vi "SPIEngineSOM.vi"(7 "NumNodes":u8=1) -> ()   [LabVIEW 2014, in "IO Node Logic Template_SPIBus0.lvlib"]
uses:
  IO Node Logic Template_SPIBus0.lvlib
  <vilib>/SPIAPI/DIO/SPI Digital IO Lines.ctl
  <vilib>/SPIAPI/DIO/SPI DIO Enable Lines.ctl
  Node/Controls/NodeResources FIFOs.ctl
  Controls/All Nodes Resources.ctl
  <vilib>/Platform/TimedLoop/XDataNode/XDataNode.xnode
  <vilib>/Platform/TimedLoop/XDataNode/nitl_modes.ctl
  <vilib>/Platform/TimedLoop/XDataNode/XDNodeRunTimeDep.lvlib
  <vilib>/Platform/TimedLoop/XDataNode/wakeup.ctl
  <vilib>/Platform/TimedLoop/XDataNode/timing_clust.ctl
  <userlib>/_NI SPI IP/FPGA/Controllers/Public/Spi Master Outputs.ctl
  <userlib>/_NI SPI IP/FPGA/Controllers/NI SPI IP FPGA.lvlib
panel:
  out "spi output":T1
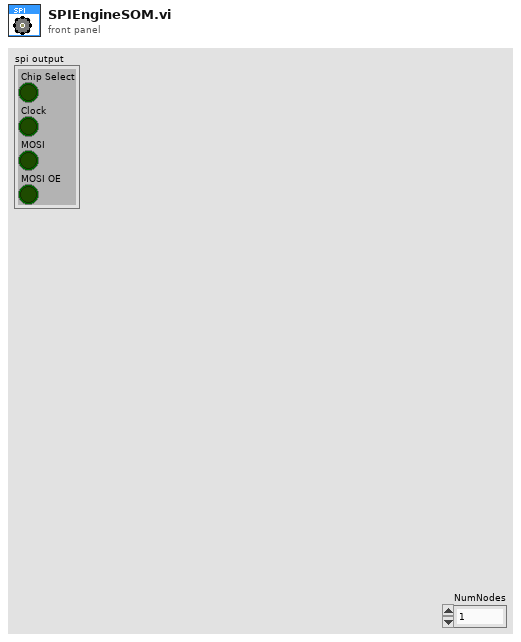
[diagram p1: front panel]
types:
  T1 = typedef "NI SPI IP FPGA.lvlib/Spi Master Outputs.ctl" = cluster{"Chip Select":bool, "Clock":bool, "MOSI":bool, "MOSI OE":bool}
  T2 = typedef "IO Node Logic Template_SPIBus0.lvlib/All Nodes Resources.ctl" = cluster{"FIFOs.Node 0":T3}
  T3 = typedef "IO Node Logic Template_SPIBus0.lvlib/NodeResources FIFOs.ctl" = cluster{"SendCmdFIFO":refnum<k21>, "ReceiveDataFIFO":refnum<k21>}
  T4 = typedef "SPI DIO Enable Lines.ctl" = cluster{"SCLK_en":refnum<k21>, "MISO_en":refnum<k21>, "MOSI_en":refnum<k21>, "CS0_en":refnum<k21>, "CS1_en":refnum<k21>, "CS2_en":refnum<k21>, "CS3_en":refnum<k21>, "CS4_en":refnum<k21>, "CS5_en":refnum<k21>}
  T5 = typedef "SPI Digital IO Lines.ctl" = cluster{"SCLK":refnum<k21>, "MISO":refnum<k21>, "MOSI":refnum<k21>, "CS 0":refnum<k21>, "CS 1":refnum<k21>, "CS 2":refnum<k21>, "CS 3":refnum<k21>, "CS 4":refnum<k21>, "CS 5":refnum<k21>}
  T6 = typedef "Internal Data (SPI API).ctl" = cluster{"DLU To SPI Engine Data FIFO":refnum<k21>, "SPI Engine to DLU Data FIFO":refnum<k21>, "Data to SPI Engine (Cache) Register":refnum<k21>, "SPI PHY Settings to SPI Engine (Cahche) Register":refnum<k21>}
  T7 = typedef "XDNodeRunTimeDep.lvlib/timing_clust.ctl" = cluster{"Expected End [f-1]":u64, "Actual End [f-1]":u64, "Finished Late? [f-1]":bool, "Expected End [i-1]":u64, "Actual End [i-1]":u64, "Finished Late? [i-1]":bool, "Expected Start [i]":u64, "Actual Start [i]":u64, "Expected Start [f]":u64, "Actual Start [f]":u64, "Source Name":string, "Structure Name":string, "Period":i64, "Deadline":i64, "Offset":i64, "Start":i64, "Priority":i32, "Timeout":i32, "Mode":T8, "Wakeup Reason":T9, "Error":errorcluster, "Source Type":string, "Secondary Source Type":string, "Global End Time":u64, "Global Start Time":u64, "Frame Duration":u64, "Iteration Duration":u64, "Assigned CPU":i32, "I/O Scan Engine Mode":u32}
  T8 = typedef "XDNodeRunTimeDep.lvlib/nitl_modes.ctl" = enum32{"No Change", "Process missed periods, maintain original phase", "Discard missed periods, maintain original phase", "Process missed periods, ignore original phase", "Discard missed periods, ignore original phase"}
  T9 = typedef "XDNodeRunTimeDep.lvlib/wakeup.ctl" = enum32{"Normal", "Aborted", "Asynchronous wakeup", "Timing source error", "Timed loop error", "Timeout"}
  T10 = typedef "IO Node Logic Template_SPIBus0.lvlib/Node_Command_Sent.ctl" = cluster{"Device ID":u8, "Data":u64, "Command":u8, "Node ID":u8, "Misc":u8}
  T11 = typedef "SPI Response Information.ctl" = cluster{"Data to Node":u64, "Node Id":u16}
  T12 = typedef "NI SPI IP FPGA.lvlib/Spi Master Inputs.ctl" = cluster{"MISO":bool}
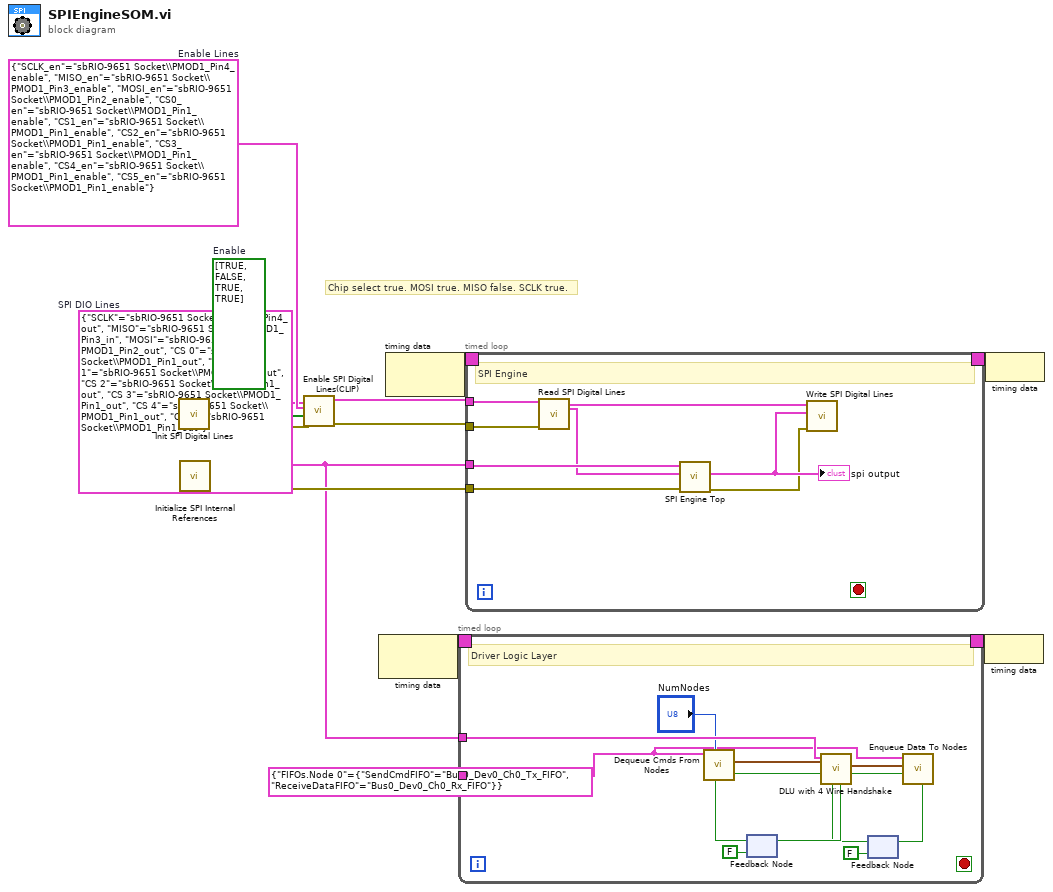
[diagram p0: block diagram]
diagram:
  w2 = bool[] [TRUE, FALSE, TRUE, TRUE]  # Enable
  w9 = T4 {"SCLK_en"="sbRIO-9651 Socket\\PMOD1_Pin4_enable", "MISO_en"="sbRIO-9651 Socket\\PMOD1_Pin3_enable", "MOSI_en"="sbRIO-9651 Socket\\PMOD1_Pin2_enable", "CS0_en"="sbRIO-9651 Socket\\PMOD1_Pin1_enable", "CS1_en"="sbRIO-9651 Socket\\PMOD1_Pin1_enable", "CS2_en"="sbRIO-9651 Socket\\PMOD1_Pin1_enable", "CS3_en"="sbRIO-9651 Socket\\PMOD1_Pin1_enable", "CS4_en"="sbRIO-9651 Socket\\PMOD1_Pin1_enable", "CS5_en"="sbRIO-9651 Socket\\PMOD1_Pin1_enable"}  # Enable Lines
  w4 = T5 {"SCLK"="sbRIO-9651 Socket\\PMOD1_Pin4_out", "MISO"="sbRIO-9651 Socket\\PMOD1_Pin3_in", "MOSI"="sbRIO-9651 Socket\\PMOD1_Pin2_out", "CS 0"="sbRIO-9651 Socket\\PMOD1_Pin1_out", "CS 1"="sbRIO-9651 Socket\\PMOD1_Pin1_out", "CS 2"="sbRIO-9651 Socket\\PMOD1_Pin1_out", "CS 3"="sbRIO-9651 Socket\\PMOD1_Pin1_out", "CS 4"="sbRIO-9651 Socket\\PMOD1_Pin1_out", "CS 5"="sbRIO-9651 Socket\\PMOD1_Pin1_out"}  # SPI DIO Lines
  # "Chip select true. MOSI true. MISO false. SCLK true."
  n1 = call <vilib>:"Init SPI Digital Lines.vi"("Chip Select DIO Lines"=w4) -> ("error out"=w12:errorcluster, "Chip Select DIO Lines"=w3:T5)  [unwired: 9 in]
  n2 = call <vilib>:"Initialize SPI Internal References.vi"() -> ("error out"=w14:errorcluster, "SPI API References"=w13:T6)  [unwired: 10 in]
  n3 = call <vilib>:"Enable SPI Digital Lines(CLIP).vi"("error in"=w12, "Enable"=w2, "Enable Lines"=w9, "SPI DIO Lines"=w3) -> ("error out"=w11:errorcluster, "Chip Select DIO Lines"=w10:T5)  [unwired: 6 in]
  n4 = node-c288() -> (w6:T7)  [unwired: 1 in]
  n5 = node-c288() -> (w8:T7)  [unwired: 1 in]
  n6 = timed-loop {
    tunnel: w13 -> [w18]
    timing: w6 -> [_]
    timing-out: [_] -> w5
    tunnel: T2 {"FIFOs.Node 0"={"SendCmdFIFO"="Bus0_Dev0_Ch0_Tx_FIFO", "ReceiveDataFIFO"="Bus0_Dev0_Ch0_Rx_FIFO"}} ("Communication FIFOs") -> [w15]
    stop <- _ stop-if-true
    # "Driver Logic Layer"
    n7 = feedback #1(FALSE ("Ready For Input?")) -> (w25:bool)
    n8 = call "Dequeue Cmds From Nodes.vi"("Ready For Output?"=w25, "NumNodes"="NumNodes", "Communication FIFOs"=w15) -> ("Cmd Received Valid"=w23:bool, "Cmd Received"=w22:T10)  [unwired: 5 in, 2 out]
    n9 = feedback #2(FALSE ("Ready for Input")) -> (w20:bool)
    n10 = call "DLU with 4 Wire Handshake.vi"("ready for output"=w20, "Input Valid"=w23, "Input Data"=w22, "Private Data In"=w18) -> ("Output Valid"=w27:bool, "Output Data"=w17:T11, "ready for Input"=w24:bool)  [unwired: 5 in]
    n11 = feedback-in #1(w24) -> ()
    n12 = call "Enqueue Data To Nodes.vi"("Input Valid"=w27, "Input Data"=w17, "Communication FIFOs"=w15) -> ("Ready for Input"=w21:bool)  [unwired: 6 in, 2 out]
    n13 = feedback-in #2(w21) -> ()
  }
  n14 = timed-loop {
    tunnel: w13 -> [w37]
    tunnel: w14 -> [w36]
    tunnel: w10 -> [w35]
    tunnel: w11 -> [w34]
    timing: w8 -> [_]
    timing-out: [_] -> w7
    stop <- _ stop-if-true
    # "SPI Engine"
    n15 = call <vilib>:"Read SPI Digital Lines.vi"("Chip Select DIO Lines"=w35, "error in"=w34) -> ("Chip Select DIO Lines Out"=w33:T5, "SPI Read Data"=w31:T12)  [unwired: 11 in, 1 out]
    n16 = call <vilib>:"SPI Engine Top.vi"("error in"=w36, "SPI Read Data"=w31, "SPI API References"=w37) -> ("error out"=w30:errorcluster, "SPI DIO Output"=w32:T1)  [unwired: 5 in, 2 out]
    "spi output" <- w32
    n17 = call <vilib>:"Write SPI Digital Lines.vi"("error in"=w30, "spi output"=w32, "Chip Select DIO Lines"=w33) -> ()  [unwired: 7 in, 2 out]
  }
  n18 = node-c288(w5) -> ()
  n19 = node-c288(w7) -> ()
